vi "Move SC Motor (SubVI).vi"(0 "String":string, 1 "Speed":i32, 2 "error out":errorcluster, 3 "Button":refnum<vi>, 4 "VISA resource name out":refnum<visa-resource-name>, 5 "Steps":refnum<vi>, 6 "Output":refnum<vi>, 7 "Input":refnum<vi>) -> ()   [LabVIEW 2013]
panel:
  out "TL Test":bool
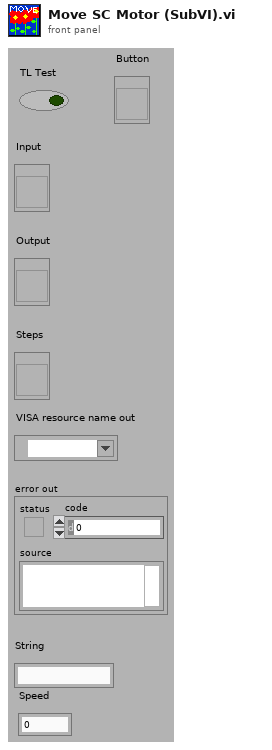
[diagram p1: front panel]
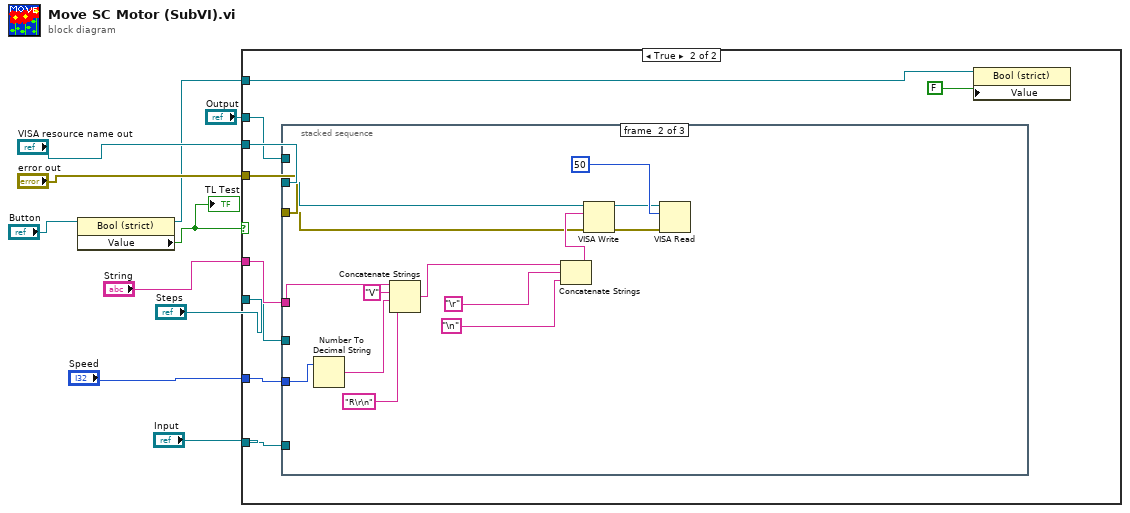
[diagram p0: block diagram]
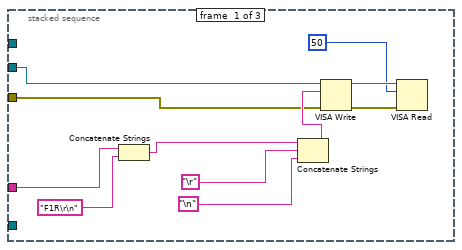
[diagram p3: hidden frame]
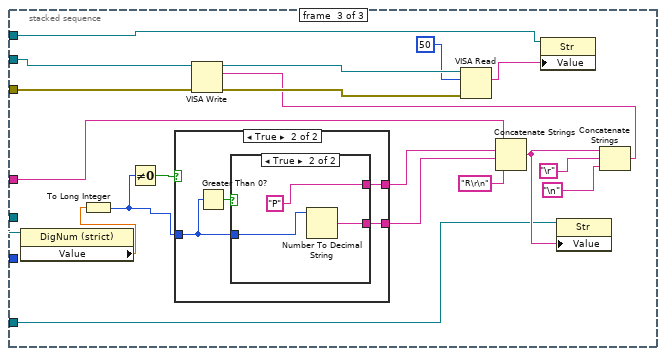
[diagram p4: hidden frame]
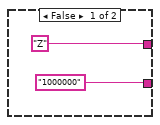
[diagram p5: hidden frame]
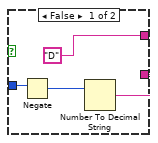
[diagram p6: hidden frame]
diagram:
  n1 = property class="Bool (strict)"(reference="Button") -> (reference out=w2:refnum<vi>, "Value"=w3:bool)  [unwired: 1 in, 1 out]
  "TL Test" <- w3
  n2 = case shown="True" w3 {
    tunnel: "VISA resource name out" -> [_ w19]
    tunnel: "error out" -> [_ w18]
    tunnel: "String" -> [_ w17]
    tunnel: "Input" -> [_ w16]
    tunnel: "Output" -> [_ w15]
    tunnel: "Steps" -> [_ w14]
    tunnel: w2 -> [_ w12]
    tunnel: "Speed" -> [_ w11]
    frame False {
    }
    frame True {
      n3 = stacked-sequence {
        tunnel: w19 -> [w24 w37 w58]
        tunnel: w18 -> [w23 w38 w57]
        tunnel: w17 -> [w22 w33 w56]
        tunnel: w16 -> [_ _ w52]
        tunnel: w15 -> [_ _ w51]
        tunnel: w14 -> [_ _ w50]
        tunnel: w11 -> [_ w34 _]
        frame #0 {
          n4 = Concatenate Strings(w22, "F1R\r\n") -> (w20:string)
          n5 = Concatenate Strings(w20, "\r", "\n") -> (w27:string)
          n6 = VISA Write(VISA resource name=w24, write buffer=w27, error in (no error)=w23) -> (VISA resource name out=w29:refnum<visa-resource-name>, error out=w30:errorcluster)  [unwired: 1 out]
          n7 = VISA Read(VISA resource name=w29, byte count=u32 50, error in (no error)=w30) -> ()  [unwired: 4 out]
        }
        frame #1 {
          n8 = Number To Decimal String(number=w34) -> (decimal integer string=w31:string)  [unwired: 1 in]
          n9 = Concatenate Strings(w33, "V" ("string"), w31, "R\r\n") -> (w35:string)
          n10 = Concatenate Strings(w35, "\r", "\n") -> (w42:string)
          n11 = VISA Write(VISA resource name=w37, write buffer=w42, error in (no error)=w38) -> (VISA resource name out=w40:refnum<visa-resource-name>, error out=w39:errorcluster)  [unwired: 1 out]
          n12 = VISA Read(VISA resource name=w40, byte count=u32 50, error in (no error)=w39) -> ()  [unwired: 4 out]
        }
        frame #2 {
          n13 = property class="DigNum (strict)"(reference=w50) -> ("Value"=w47:dbl)  [unwired: 1 in, 2 out]
          n14 = To Long Integer(number=w47) -> (32bit integer=w45:i32)
          n15 = Not Equal To 0?(x=w45) -> (x != 0?=w46:bool)
          n16 = case shown="True" w46 {
            tunnel: ["Z" w70] -> w49
            tunnel: ["1000000" w69] -> w48
            tunnel: w45 -> [_ w67]
            frame False {
            }
            frame True {
              n17 = Greater Than 0?(x=w67) -> (x > 0?=w68:bool)
              n18 = case shown="True" w68 {
                tunnel: ["D" ("string") "P" ("string")] -> w70
                tunnel: [w71 w76] -> w69
                tunnel: w67 -> [w73 w75]
                frame False {
                  n19 = Negate(x=w73) -> (-x=w72:i32)
                  n20 = Number To Decimal String(number=w72) -> (decimal integer string=w71:string)  [unwired: 1 in]
                }
                frame True {
                  n21 = Number To Decimal String(number=w75) -> (decimal integer string=w76:string)  [unwired: 1 in]
                }
              }
            }
          }
          n22 = Concatenate Strings(w56, w49, w48, "R\r\n" ("string")) -> (w54:string)
          n23 = property class="Str"(reference=w52, "Value"=w54) -> ()  [unwired: 1 in, 2 out]
          n24 = Concatenate Strings(w54, "\r", "\n") -> (w61:string)
          n25 = VISA Write(VISA resource name=w58, write buffer=w61, error in (no error)=w57) -> (VISA resource name out=w63:refnum<visa-resource-name>, error out=w64:errorcluster)  [unwired: 1 out]
          n26 = VISA Read(VISA resource name=w63, byte count=u32 50, error in (no error)=w64) -> (read buffer=w53:string)  [unwired: 3 out]
          n27 = property class="Str"(reference=w51, "Value"=w53) -> ()  [unwired: 1 in, 2 out]
        }
      }
      n28 = property class="Bool (strict)"(reference=w12, "Value"=FALSE) -> ()  [unwired: 1 in, 2 out]
    }
  }
